vi "IsTransitionComplete.vi"(4 "Cutoff Range For Completion (deg)":i32=10, 5 "Trusted Absolute Wind (deg)":dbl, 6 "Last Commanded Regime":T1, 7 "Altered regime boundaries":T2=[0, 70, 140, 180, 220, 290], 8 "Current Regime":T1, 9 "Desired Regime":T1, 10 "Desired Heading (deg)":dbl, 11 "Robot Heading (deg)":dbl) -> (3 "Is Transition Complete?":bool)   [LabVIEW 2013]
doc: "This VI should check whether the boat's current transition is complete, and should probably do so by comparing the desired heading to the boat's actual heading. Once the two are within some error bound, this VI returns 'TRUE' and tells the boat the turn is over.\n\nIf the commanded regime is not adjacent to the desired regime (e.g. we are tacking but we want to end in the reach regime, not the upwind regime) then this VI considers the center of the upwind regime as the new desired heading and checks off the tack transition. At that boat the code above this should say \"I'm in Upwind and want to be reaching, I'm going to command the next transition state\". This way the boat will switch transition states as it goes around the circle seen in https://docs.google.com/file/d/0B6St7IDGiYunU3FLWTZHTUFHWHc/edit?usp=drive_web\n\nEric Schneider, Feb. 2014"
uses:
  Data/TypeDefs/Sailing Regimes.ctl
  Data/TypeDefs/Regime Boundaries.ctl
  Utilities/Math/Angles/Angle/Angle.lvclass
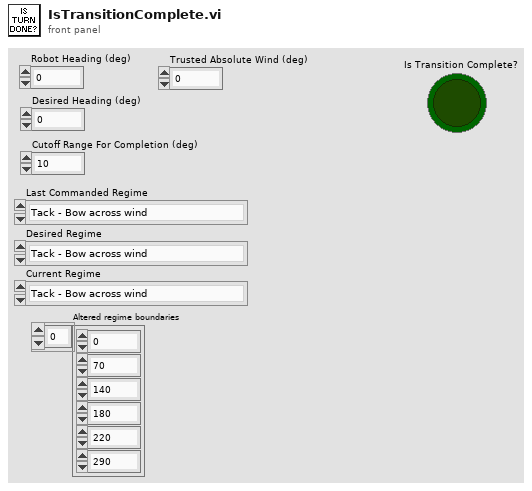
[diagram p1: front panel]
types:
  T1 = typedef "Sailing Regimes.ctl" = enum16{"Tack - Bow across wind", "Upwind - Starboard Tack", "Turn between Upwind/Reach - Starboard Tack", "Reach - Starboard Tack", "Turn between Reach/Run - Starboard Tack", "Run - Starboard Tack", "Jibe - Stern across wind", "Run - Port Tack", "Turn between Reach/Run - Port Tack", "Reach - Port Tack", "Turn between Upwind/Reach - Port Tack", "Upwind - Port Tack"}
  T2 = typedef "Regime Boundaries.ctl" = i32[]
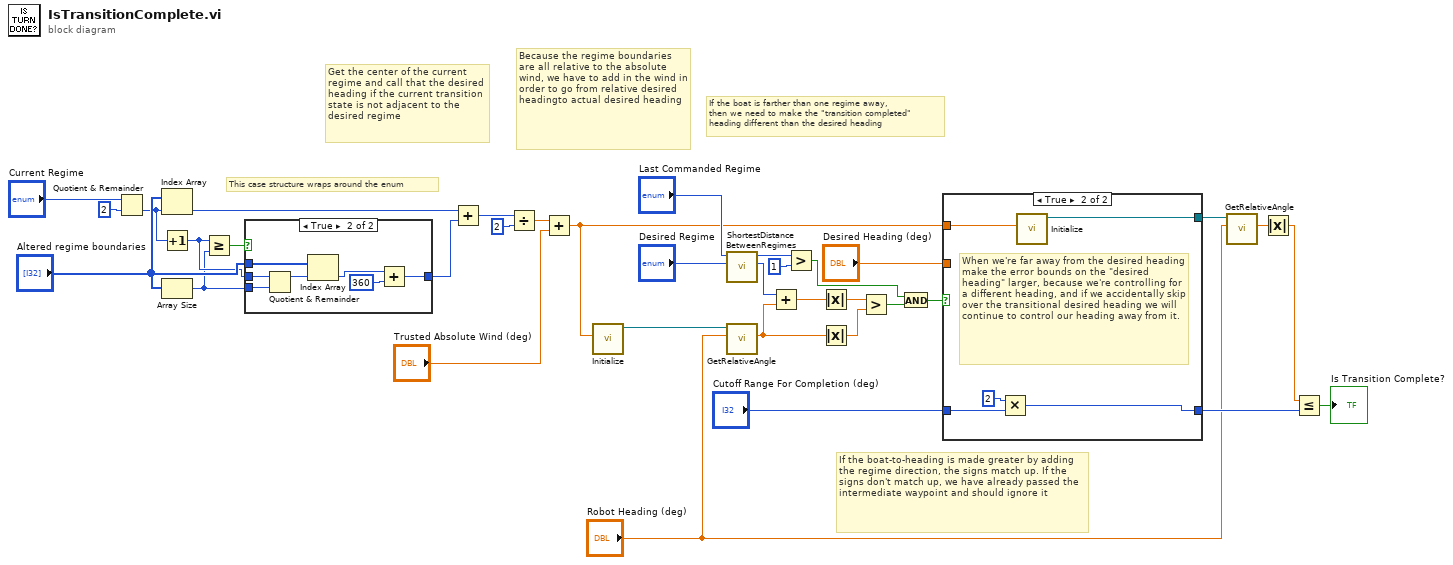
[diagram p0: block diagram]
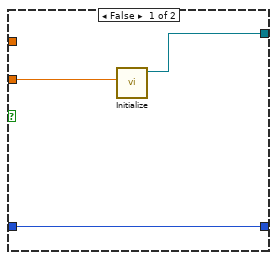
[diagram p2: hidden frame]
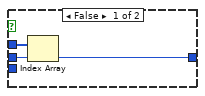
[diagram p3: hidden frame]
diagram:
  # "If the boat-to-heading is made greater by adding the regime direction, the signs match up. If the signs don't match up, we have already passed the intermediate waypoint and should ignore it"
  # "Because the regime boundaries are all relative to the absolute wind, we have to add in the wind in order to go from relative desired headingto actual desired heading"
  # "This case structure wraps around the enum"
  # "Get the center of the current regime and call that the desired heading if the current transition state is not adjacent to the desired regime"
  # "If the boat is farther than one regime away,\nthen we need to make the \"transition completed\"\nheading different than the desired heading"
  n1 = Quotient & Remainder(x="Current Regime", y=2) -> (floor(x/y)=w26:i32)  [unwired: 1 out]
  n2 = Index Array(array="Altered regime boundaries", index=w26) -> (element=w20:i32)
  n3 = Increment(x=w26) -> (x+1=w24:i32)
  n4 = Array Size(array="Altered regime boundaries") -> (size(s)=w23:i32)
  n5 = Greater Or Equal?(x=w24, y=w23) -> (x >= y?=w25:bool)
  n6 = case shown="True" w25 {
    tunnel: "Altered regime boundaries" -> [w38 w45]
    tunnel: w24 -> [w37 w43]
    tunnel: w23 -> [_ w42]
    tunnel: [w36 w39] -> w21
    frame False {
      n7 = Index Array(array=w38, index=w37) -> (element=w36:i32)
    }
    frame True {
      n8 = Quotient & Remainder(x=w43, y=w42) -> (x-y*floor(x/y)=w41:i32)  [unwired: 1 out]
      n9 = Index Array(array=w45, index=w41) -> (element=w44:i32)
      n10 = Add(x=w44, y=360) -> (x+y=w39:i32)
    }
  }
  n11 = Add(x=w20, y=w21) -> (x+y=w22:i32)
  n12 = Divide(x=w22, y=2) -> (x/y=w18:dbl)
  n13 = Add(x=w18, y="Trusted Absolute Wind (deg)") -> (x+y=w7:dbl)
  n14 = call "Initialize.vi"("Input Angle (Deg.)"=w7) -> ("Angle out"=w6:refnum<class "Angle.lvclass">)  [unwired: 9 in, 1 out]
  n15 = call "ShortestDistanceBetweenRegimes.vi"("Regime 2"="Desired Regime", "Regime 1"="Last Commanded Regime") -> ("Direction to Regime 2"=w10:i32, "Distance between the two regimes"=w17:i32)  [unwired: 8 in]
  n16 = call "GetRelativeAngle.vi"("Boat Heading (Deg.)"="Robot Heading (deg)", "Angle in"=w6) -> ("Relative Angle"=w5:dbl)  [unwired: 7 in, 2 out]
  n17 = Add(x=w10, y=w5) -> (x+y=w9:dbl)
  n18 = Greater?(x=w17, y=1) -> (0:w16:bool)
  n19 = Absolute Value(x=w9) -> (abs(x)=w4:dbl)
  n20 = Absolute Value(x=w5) -> (abs(x)=w3:dbl)
  n21 = Greater?(x=w4, y=w3) -> (0:w2:bool)
  n22 = And(x=w16, y=w2) -> (x .and. y?=w14:bool)
  n23 = case shown="True" w14 {
    tunnel: [w47 w50] -> w11
    tunnel: "Cutoff Range For Completion (deg)" -> [w48 w52]
    tunnel: [w48 w51] -> w12
    tunnel: w7 -> [_ w49]
    tunnel: "Desired Heading (deg)" -> [w46 _]
    frame False {
      n24 = call "Initialize.vi"("Input Angle (Deg.)"=w46) -> ("Angle out"=w47:refnum<class "Angle.lvclass">)  [unwired: 9 in, 1 out]
    }
    frame True {
      # "When we're far away from the desired heading make the error bounds on the \"desired heading\" larger, because we're controlling for a different heading, and if we accidentally skip over the transitional desired heading we will continue to control our heading away from it."
      n25 = Multiply(x=2, y=w52) -> (x*y=w51:i32)
      n26 = call "Initialize.vi"("Input Angle (Deg.)"=w49) -> ("Angle out"=w50:refnum<class "Angle.lvclass">)  [unwired: 9 in, 1 out]
    }
  }
  n27 = call "GetRelativeAngle.vi"("Boat Heading (Deg.)"="Robot Heading (deg)", "Angle in"=w11) -> ("Relative Angle"=w35:dbl)  [unwired: 7 in, 2 out]
  n28 = Absolute Value(x=w35) -> (abs(x)=w34:dbl)
  n29 = Less Or Equal?(x=w34, y=w12) -> (x <= y?=→"Is Transition Complete?":bool)
